vi "Lambda_tau,T,W(s).vi"(8 "W":dbl, 9 "T":dbl, 10 "t":dbl, 11 "s":dbl) -> (3 "L_tau,T,W(s)":dbl)   [LabVIEW 2021, in "Phasor.lvlib"]
uses:
  Phasor/Phasor.lvlib
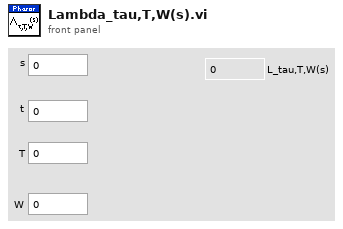
[diagram p1: front panel]
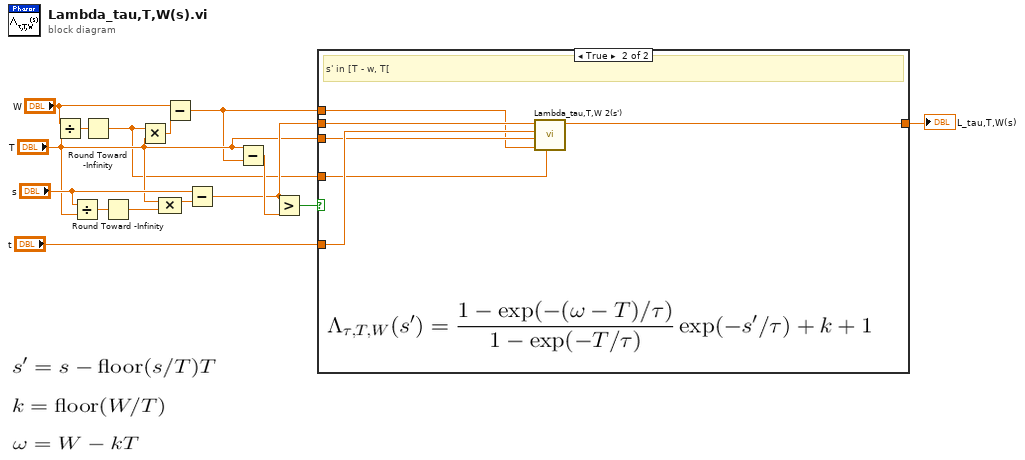
[diagram p0: block diagram]
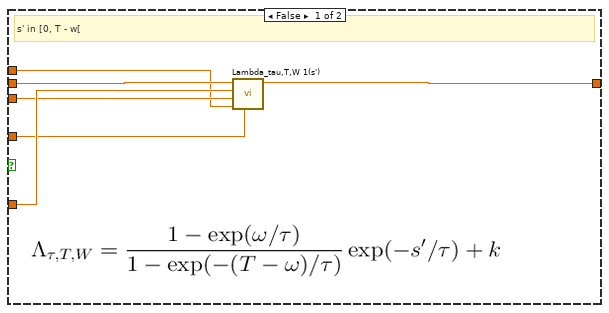
[diagram p2: hidden frame]
diagram:
  n1 = Divide(x="W", y="T") -> (x/y=w12:dbl)
  n2 = Divide(x="s", y="T") -> (x/y=w14:dbl)
  n3 = Round Toward -Infinity(1:w12) -> (0:w2:dbl)
  n4 = Round Toward -Infinity(1:w14) -> (0:w9:dbl)
  n5 = Multiply(x=w2, y="T") -> (x*y=w11:dbl)
  n6 = Compound Arithmetic op=MULTIPLY("T", w9) -> (w15:dbl)
  n7 = Subtract(x="W", y=w11) -> (x-y=w3:dbl)
  n8 = Subtract(x="s", y=w15) -> (x-y=w6:dbl)
  n9 = Subtract(x="T", y=w3) -> (x-y=w8:dbl)
  n10 = Greater?(x=w6, y=w8) -> (0:w7:bool)
  n11 = case shown="True" w7 {
    tunnel: w6 -> [w21 w27]
    tunnel: "t" -> [w19 w26]
    tunnel: "T" -> [w18 w25]
    tunnel: w3 -> [w17 w24]
    tunnel: w2 -> [w16 w23]
    tunnel: [w20 w22] -> w1
    frame False {
      # "s' in [0, T - w["
      n12 = call "Lambda_tau,T,W 1(s').vi"("k"=w16, "w"=w17, "T"=w18, "t"=w19, "s'"=w21) -> ("L_t,T,W(s')"=w20:dbl)  [unwired: 6 in]
    }
    frame True {
      # "s' in [T - w, T["
      n13 = call "Lambda_tau,T,W 2(s').vi"("k"=w23, "w"=w24, "T"=w25, "t"=w26, "s'"=w27) -> ("L_t,T,W(s')"=w22:dbl)  [unwired: 6 in]
    }
  }
  "L_tau,T,W(s)" <- w1
